vi "Set Exposure Time.vi"(8 "error in (no error)":errorcluster, 11 "CCDCamera in":refnum<class "iKon-L.lvclass">) -> (0 "error out":errorcluster, 3 "CCDCamera out":refnum<class "iKon-L.lvclass">)   [LabVIEW 2018, in "iKon-L.lvclass"]
doc: "Set the exposure time in seconds"
uses:
  iKon-L.lvclass
  C:/Users/Denis/Desktop/S4ACS/S4ACS/Sim_CCD/Sim_CCD.lvclass
  Sim_CCD/Sim_CCD.lvclass
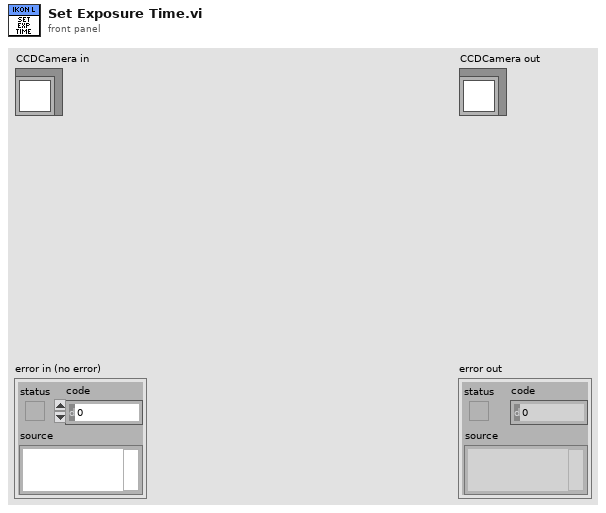
[diagram p1: front panel]
types:
  T1 = cluster{"EXPTIME":dbl, "#FRAMES":u32, "COOLER_POWER_STATUS":u16, "TEMP":i32}
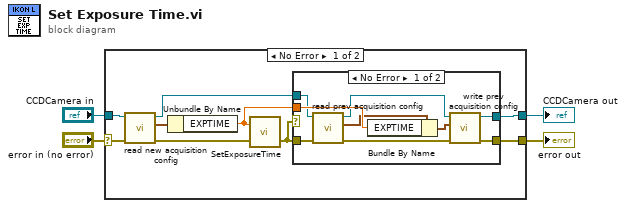
[diagram p0: block diagram]
diagram:
  n1 = case shown="No Error" "error in (no error)" {
    selector: "error in (no error)" -> [w9 w25]
    tunnel: "CCDCamera in" -> [w8 w26]
    tunnel: [w13 w25] -> w2
    tunnel: [w5 w26] -> w1
    frame No Error {
      n2 = call "read new acquisition config.vi"("error in (no error)"=w9, "Simulated_CCD_Camera in"=w8) -> ("error out"=w7:errorcluster, "new acquisition configuration"=w10:T1, "Simulated_CCD_Camera out"=w6:refnum<class "iKon-L.lvclass">)  [unwired: 7 in]
      n3 = Unbundle By Name(w10) -> ("EXPTIME"=w12:dbl)
      n4 = call <userlib>:"SetExposureTime.vi"("error in (no error)"=w7, "time"=w12) -> ("error out"=w11:errorcluster)  [unwired: 1 out]
      n5 = case shown="No Error" w11 {
        tunnel: [w14 w24] -> w13
        tunnel: w11 -> [w21 w24]
        tunnel: w12 -> [w22 _]
        tunnel: w6 -> [w20 w23]
        tunnel: [w15 w23] -> w5
        frame No Error {
          n6 = call "read prev acquisition config.vi"("error in (no error)"=w21, "Simulated_CCD_Camera in"=w20) -> ("error out"=w19:errorcluster, "prev acquisition configuration"=w17:T1, "Simulated_CCD_Camera out"=w16:refnum<class "iKon-L.lvclass">)  [unwired: 7 in]
          n7 = Bundle By Name(cluster=w17, "EXPTIME"=w22) -> (w18:T1)
          n8 = call "write prev acquisition config.vi"("error in (no error)"=w19, "prev acquisition configuration"=w18, "Simulated_CCD_Camera in"=w16) -> ("error out"=w14:errorcluster, "Simulated_CCD_Camera out"=w15:refnum<class "iKon-L.lvclass">)  [unwired: 7 in]
        }
        frame Error {
        }
      }
    }
    frame Error {
    }
  }
  "error out" <- w2
  "CCDCamera out" <- w1
